vi "RT Driver VI.vi"(7 "Operation":T1, 11 "Device Reference in":T2 format="%.0x") -> (0 "Error Code":i32)   [LabVIEW 2019, in "Ghost Bus Addon Engine.lvlib"]
uses:
  Ghost Bus Addon Engine.lvlib
  <vilib>/NI VeriStand/Custom Device API/Custom Device Item Ref.ctl
  <vilib>/NI VeriStand/Custom Device API/Hardware Interface Driver VI Operation.ctl
  Addon Shared/Types/Exported.OnCompile.ctl
  Addon Shared/Types/XNET Settings.ctl
  Addon Shared/Types/XNET Port Settings.ctl
  Addon Shared/Types/Exported.Bus.Settings.ctl
  Addon Shared/Types/Exported.Frames.Settings.ctl
  Addon Shared/Types/Frame Settings.ctl
  <vilib>/NI/NIVS Inline Async API/_VS Inline Async API/VS Inline Async API/Types/Error Handling Settings.ctl
  <vilib>/NI/NIVS Inline Async API/_VS Inline Async API/VS Inline Async API/VS Inline Async API.lvclass
  <vilib>/NI/NIVS Inline Async API/_VS Inline Async API/VS Inline Async API/VS Inline Async API.lvclass/VS Inline Async API.ctl
  <vilib>/NI/NIVS Inline Async API/_Data Access Engine/Data Access Engine/Data Access Engine.lvclass/Data Access Engine.ctl
  <vilib>/NI/NIVS Inline Async API/_Data Access Engine/Access Type Classes/Write/Write.lvclass/Write.ctl
  <vilib>/NI/NIVS Inline Async API/_Data Access Engine/Access Type Classes/ReadWrite/ReadWrite.lvclass/ReadWrite.ctl
  <vilib>/NI/NIVS Inline Async API/_Data Access Engine/Access Type Classes/Read/Read.lvclass/Read.ctl
  <vilib>/NI/NIVS Inline Async API/_Data Access Engine/Data Access Engine/Methods/Data.Engine.Read Data from HW.vi
  <vilib>/NI/NIVS Inline Async API/_VS Inline Async API/Error Handling Process/SubVIs/Error.GetError.vi
  <vilib>/NI/NIVS Inline Async API/_Data Access Engine/Data Access Engine/Methods/Data.Engine.Write Data to HW.vi
  <vilib>/NI/NIVS Inline Async API/_Data Access Engine/Access Type Classes/ReadWrite/ReadWrite.EngineData.vi
  <vilib>/NI/NIVS Inline Async API/_Data Access Engine/Access Type Classes/Write/Write.EngineData.vi
  <vilib>/NI/NIVS Inline Async API/_Data Access Engine/Access Type Classes/Read/Read.EngineData.vi
  <vilib>/NI VeriStand/Custom Device API/NI VeriStand - Get Channel Value by Data Reference.vi
  <vilib>/NI VeriStand/Custom Device API/NI VeriStand - Set Channel Value by Data Reference.vi
  <vilib>/NI VeriStand/Custom Device API/NI VeriStand - Get Channel Values by Block Data Reference.vi
  Addon Shared/SubVIs/GUID Lookup.vi
  <vilib>/NI VeriStand/Custom Device API/Get Item Property (Variant).vi
  <vilib>/Utility/SystemLogging/Write to System Log.vi
  <vilib>/NI VeriStand/Custom Device API/Global Data Refs.vi
  <vilib>/NI VeriStand/Custom Device API/Custom Device API.lvlib
  Addon Shared/Ghost Bus Addon Shared.lvlib
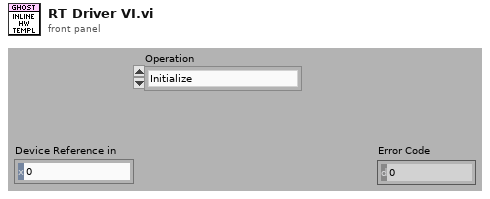
[diagram p1: front panel]
types:
  T1 = typedef "Custom Device API.lvlib/Hardware Interface Driver VI Operation.ctl" = enum16{"Initialize", "Start", "Read Data from HW", "Write Data to HW", "Close"}
  T2 = typedef "Custom Device API.lvlib/Custom Device Item Ref.ctl" = u64
  T3 = cluster{"Process":refnum<class "VS Inline Async API.lvclass">, "Name":string}
  T4 = typedef "VS Inline Async API.lvlib/VS Inline Async API.lvclass/Error Handling Settings.ctl" = cluster{"Write to SystemLog (F)":bool}
  T5 = typedef "Ghost Bus Addon Shared.lvlib/Exported.OnCompile.ctl" = cluster{"Name":string, "XNET Settings":T6, "To Primary Info":T8, "To Ghost Info":T8}
  T6 = typedef "Ghost Bus Addon Shared.lvlib/XNET Settings.ctl" = cluster{"Database":refnum<k21>, "Cluster":refnum<k21>, "Primary":T7, "Ghost":T7}
  T7 = typedef "Ghost Bus Addon Shared.lvlib/XNET Port Settings.ctl" = cluster{"Port":string, "Baud Rate":u64, "Termination":u32, "CAN I/O Mode":u32, "FD Baud Rate":u64, "Priority":i32, "FD ISO Mode":u32}
  T8 = typedef "Ghost Bus Addon Shared.lvlib/Exported.Bus.Settings.ctl" = cluster{"Name":string, "Overrides?":bool, "Frames":T9[]}
  T9 = typedef "Ghost Bus Addon Shared.lvlib/Exported.Frames.Settings.ctl" = cluster{"Name":string, "Frame.Settings":T10, "Length":i32, "Offset":i32, "Signals":string[]}
  T10 = typedef "Ghost Bus Addon Shared.lvlib/Frame Settings.ctl" = cluster{"ID":u32}
  T11 = typedef "Ghost Bus Addon Engine.lvlib/RT Bus Settings.ctl" = cluster{"Name":string, "Overrides?":bool, "XNET Refs":T12, "Port Info":T7, "Frames":variant}
  T12 = typedef "Ghost Bus Addon Engine.lvlib/RT XNET Refs.ctl" = cluster{"Incoming":refnum<k21>, "Outgoing":refnum<k21>}
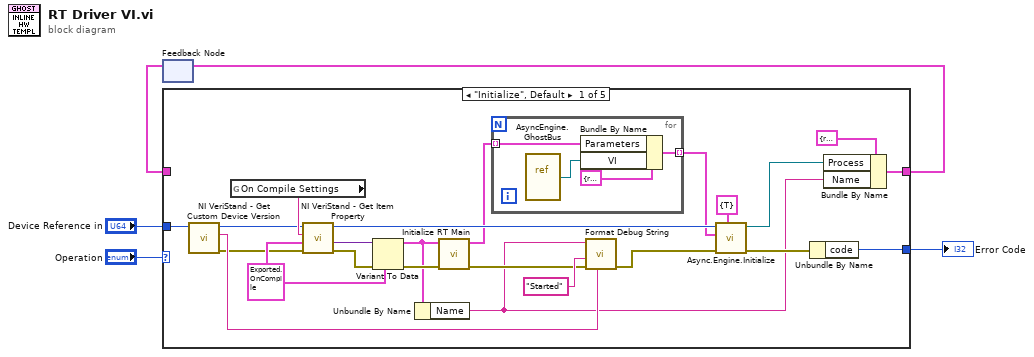
[diagram p0: block diagram]
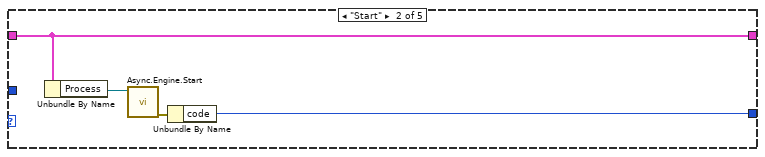
[diagram p2: hidden frame]
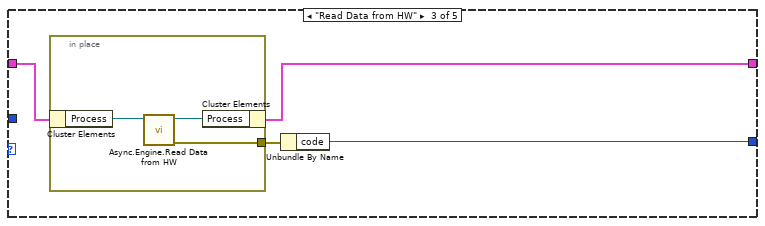
[diagram p3: hidden frame]
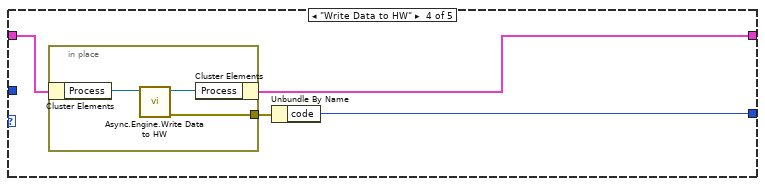
[diagram p4: hidden frame]
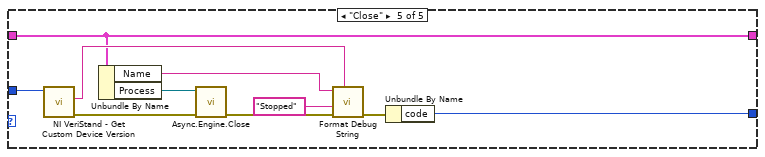
[diagram p5: hidden frame]
diagram:
  n1 = feedback #1() -> (w3:T3)  [unwired: 1 out]
  n2 = case shown="\"Initialize\", Default" "Operation" {
    tunnel: [w27 w33 w39 w47 w51] -> w4
    tunnel: w3 -> [_ w33 w40 w46 w51]
    tunnel: [w28 w36 w37 w44 w56] -> w2
    tunnel: "Device Reference in" -> [w26 _ _ _ w60]
    frame "Initialize", Default {
      w21 = T5 {"Name"="", "XNET Settings"={"Database"="", "Cluster"="", "Primary"={"Port"="", "Baud Rate"=500000, "Termination"=1, "CAN I/O Mode"=0, "FD Baud Rate"=500000, "Priority"=100, "FD ISO Mode"=0}, "Ghost"={"Port"="", "Baud Rate"=0, "Termination"=0, "CAN I/O Mode"=0, "FD Baud Rate"=500000, "Priority"=100, "FD ISO Mode"=0}}, "To Primary Info"={"Name"="", "Overrides?"=FALSE, "Frames"=[]}, "To Ghost Info"={"Name"="", "Overrides?"=FALSE, "Frames"=[]}} ("Cluster")
      n3 = call <vilib>:"NI VeriStand - Get Custom Device Version.vi"("Device Ref in"=w26) -> ("error out"=w9:errorcluster, "Value"=w17:string, "Device Ref out"=w8:T2)  [unwired: 8 in]
      n4 = global read "GUID Lookup.vi" "On Compile Settings"() -> (w24:string)
      n5 = call-poly <vilib>:"NI VeriStand - Get Item Property.vi"("error in (no error)"=w9, "Default Value"=w21, "Property Name"=w24, "Item Ref in"=w8) -> ("error out"=w22:errorcluster, "Value"=w23:variant, "Item Ref out"=w20:T2)  [unwired: 4 in, 1 out]
      n6 = Variant To Data(error in=w22, type=w21, Variant=w23) -> (data=w7:T5, error out=w12:errorcluster)
      n7 = Unbundle By Name(w7) -> ("Name"=w6:string)
      n8 = call "Initialize RT Main.vi"("error in (no error)"=w12, "OnCompile Settings"=w7) -> ("error out"=w13:errorcluster, "Settings"=w10:T11[])  [unwired: 8 in]
      n9 = for {
        tunnel: [w31] -> w11 mode=indexing
        tunnel: w10 -> [w29] mode=indexing
        n10 = vi-ref "AsyncEngine.GhostBus.vi"() -> (w30:refnum<vi>)
        n11 = Bundle By Name(cluster=cluster{"VI":refnum<vi>, "Parameters":variant} {"VI"=refnum, "Parameters"=variant} ("Process"), "Parameters"=w29, "VI"=w30) -> (w31:cluster{"VI":refnum<vi>, "Parameters":variant})
      }
      n12 = call "Format Debug String.vi"("Version"=w17, "error in (no error)"=w13, "State"="Started", "Name"=w6) -> ("error out"=w15:errorcluster)  [unwired: 7 in]
      n13 = call <vilib>:"Async.Engine.Initialize.vi"("Error Log Settings"=T4 {"Write to SystemLog (F)"=TRUE}, "error in (no error)"=w15, "Processes"=w11, "Custom Device Ref"=w20) -> ("error out"=w16:errorcluster, "Async"=w25:refnum<class "VS Inline Async API.lvclass">)  [unwired: 6 in]
      n14 = Unbundle By Name(w16) -> ("code"=w28:i32)
      n15 = Bundle By Name(cluster=T3 {"Process"=refnum, "Name"=""} ("input cluster"), "Process"=w25, "Name"=w6) -> (w27:T3)
    }
    frame "Start" {
      n16 = Unbundle By Name(w33) -> ("Process"=w35:refnum<class "VS Inline Async API.lvclass">)
      n17 = call <vilib>:"Async.Engine.Start.vi"("VS Inline Async API in"=w35) -> ("error out"=w34:errorcluster)  [unwired: 9 in, 1 out]
      n18 = Unbundle By Name(w34) -> ("code"=w36:i32)
    }
    frame "Read Data from HW" {
      n19 = in-place {
        in-place-border: [w41] -> w38
        n20 = in-place-cluster #2(w40) -> ("Process"=w43:refnum<class "VS Inline Async API.lvclass">)
        n21 = call <vilib>:"Async.Engine.Read Data from HW.vi"("Async in"=w43) -> ("error out"=w41:errorcluster, "Async out"=w42:refnum<class "VS Inline Async API.lvclass">)  [unwired: 9 in]
        n22 = in-place-cluster #2("Process"=w42) -> (w39:T3)
      }
      n23 = Unbundle By Name(w38) -> ("code"=w37:i32)
    }
    frame "Write Data to HW" {
      n24 = in-place {
        in-place-border: [w48] -> w45
        n25 = in-place-cluster #3(w46) -> ("Process"=w50:refnum<class "VS Inline Async API.lvclass">)
        n26 = call <vilib>:"Async.Engine.Write Data to HW.vi"("VS Inline Async API in"=w50) -> ("error out"=w48:errorcluster, "VS Inline Async API out"=w49:refnum<class "VS Inline Async API.lvclass">)  [unwired: 9 in]
        n27 = in-place-cluster #3("Process"=w49) -> (w47:T3)
      }
      n28 = Unbundle By Name(w45) -> ("code"=w44:i32)
    }
    frame "Close" {
      n29 = call <vilib>:"NI VeriStand - Get Custom Device Version.vi"("Device Ref in"=w60) -> ("error out"=w58:errorcluster, "Value"=w57:string)  [unwired: 8 in, 1 out]
      n30 = Unbundle By Name(w51) -> ("Name"=w52:string, "Process"=w59:refnum<class "VS Inline Async API.lvclass">)
      n31 = call <vilib>:"Async.Engine.Close.vi"("error in (no error)"=w58, "Async in"=w59) -> ("error out"=w53:errorcluster)  [unwired: 8 in, 1 out]
      n32 = call "Format Debug String.vi"("Version"=w57, "error in (no error)"=w53, "State"="Stopped", "Name"=w52) -> ("error out"=w54:errorcluster)  [unwired: 7 in]
      n33 = Unbundle By Name(w54) -> ("code"=w56:i32)
    }
  }
  "Error Code" <- w2
  n34 = feedback-in #1(w4) -> ()
